vi "Legend2007.vi"   [LabVIEW 2013]
uses:
  <vilib>/Heliosphere Research LLC/Advanced Plotting Toolkit/api_annotations/LegendPositions.ctl
  ModeType.ctl
  <vilib>/Heliosphere Research LLC/Advanced Plotting Toolkit/api_plotting/Histogram_Automatic.vi
  <vilib>/Heliosphere Research LLC/Advanced Plotting Toolkit/Advanced Plotting Toolkit.lvlib
types:
  T1 = typedef "ModeType.ctl" = enum16{"Normal", "Expected Failure", "Skipped"}
  T2 = typedef "Advanced Plotting Toolkit.lvlib/LegendPositions.ctl" = enum16{"Default", "Top Right", "Top", "Top Left", "Left", "Bottom Left", "Bottom", "Bottom Right", "Right", "Center"}
  T3 = typedef "Advanced Plotting Toolkit.lvlib/PlotID.ctl" = i32
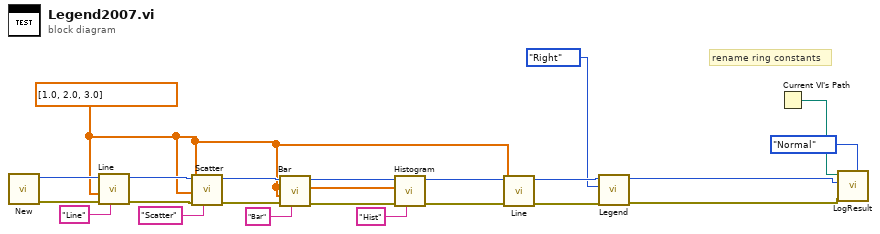
[diagram p0: block diagram]
diagram:
  w3 = dbl[] [1.0, 2.0, 3.0] ("Y Data")
  # "rename ring constants"
  n1 = call <vilib>:"New.vi"() -> ("error out"=w17:errorcluster, "Plot ID"=w21:T3)  [unwired: 10 in]
  n2 = call <vilib>:"Line.vi"("Legend Title"="Line", "error in (no error)"=w17, "Y Data"=w3, "Plot ID"=w21) -> ("error out"=w16:errorcluster, "Plot ID out"=w20:T3)  [unwired: 6 in]
  n3 = call <vilib>:"Scatter.vi"("Legend Title"="Scatter", "error in (no error)"=w16, "Y Data"=w3, "X Data"=w3, "Plot ID"=w20) -> ("error out"=w15:errorcluster, "Plot ID Out"=w19:T3)  [unwired: 5 in]
  n4 = call <vilib>:"Bar.vi"("Legend Title"="Bar", "error in (no error)"=w15, "Bar Lengths"=w3, "Plot ID"=w19) -> ("error out"=w14:errorcluster, "Plot ID Out"=w18:T3)  [unwired: 6 in]
  n5 = call-poly <vilib>:"Histogram.vi"("Legend Title"="Hist", "error in (no error)"=w14, "Data"=w3, "Plot ID"=w18) -> ("error out"=w6:errorcluster, "Plot ID Out"=w9:T3)  [unwired: 6 in]
  n6 = call <vilib>:"Line.vi"("error in (no error)"=w6, "Y Data"=w3, "Plot ID"=w9) -> ("error out"=w5:errorcluster, "Plot ID out"=w8:T3)  [unwired: 7 in]
  n7 = call <vilib>:"Legend.vi"("error in (no error)"=w5, "Position"=LegendPositions."Right", "Plot ID"=w8) -> ("error out"=w4:errorcluster, "Plot ID Out"=w7:T3)  [unwired: 7 in]
  n8 = Current VI's Path() -> (path=w22:path)
  n9 = call "LogResult.vi"("Mode"=ModeType."Normal", "Test Result"=w4, "Test Artifact"=w7, "VI Path"=w22) -> ()  [unwired: 8 in]
